vi "niDDC temp - read debug info.vi"(8 "error in (no error)":errorcluster, 11 "Class in":refnum<class "7976R_v1.lvclass">) -> (0 "error out":errorcluster, 1 "DDC":T1, 2 "FPGA":T3, 3 "Class out":refnum<class "7976R_v1.lvclass">)   [LabVIEW 2015, in "7976R_v1.lvclass"]
uses:
  <userlib>/SE-APP-Receiver/NI5772/7976R_v1/7976R_v1.lvclass
  <userlib>/SE-APP-Receiver/NI5772/7976R_v1/Private/FPGA VI Reference_DDC_v1.8.ctl
  <userlib>/SE-APP-Receiver/NI5772/7976R_v1/7976R_v1.lvclass/7976R_v1.ctl
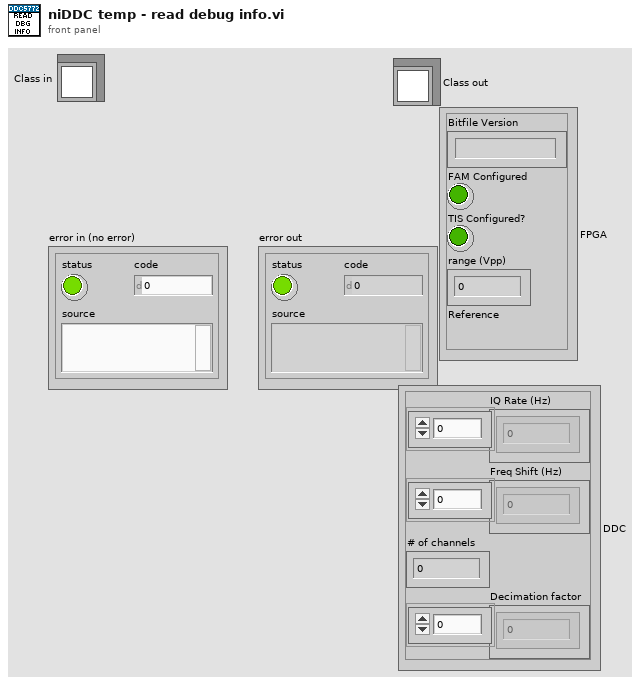
[diagram p1: front panel]
types:
  T1 = cluster{"IQ Rate (Hz)":dbl[], "Freq Shift (Hz)":dbl[], "# of channels":u8, "Decimation factor":dbl[]}
  T2 = typedef "7976R_v1.lvclass/FPGA VI Reference_DDC_v1.8.ctl" = refnum<k20>
  T3 = cluster{"Bitfile Version":string, "FAM Configured":bool, "TIS Configured?":bool, "range (Vpp)":dbl, "Reference":T2}
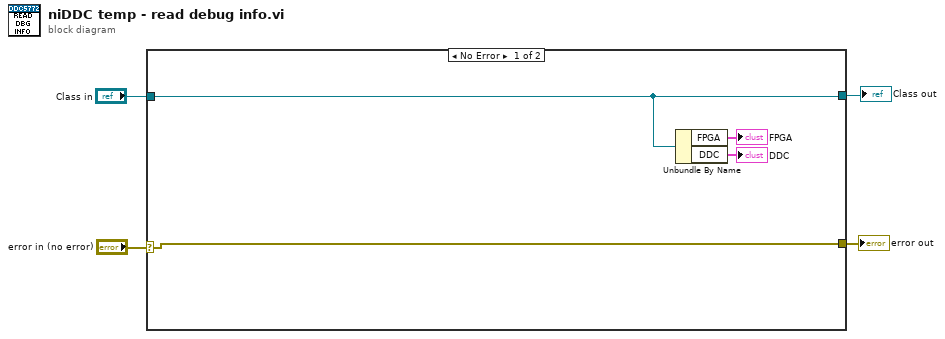
[diagram p0: block diagram]
diagram:
  n1 = case shown="No Error" "error in (no error)" {
    selector: "error in (no error)" -> [w8 w10]
    tunnel: [w8 w10] -> w4
    tunnel: "Class in" -> [w7 w9]
    tunnel: [w7 w9] -> w1
    frame No Error {
      n2 = Unbundle By Name(w7) -> ("FPGA"=→"FPGA":T3, "DDC"=→"DDC":T1)
    }
    frame Error {
    }
  }
  "error out" <- w4
  "Class out" <- w1
